vi "Write Resource Name.vi"(8 "error in (no error)":errorcluster, 10 "Resource Name":refnum<k15>, 11 "Power Meter in":refnum<class "Power Meter.lvclass">) -> (0 "error out":errorcluster, 3 "Power Meter out":refnum<class "Power Meter.lvclass">)   [LabVIEW 2023, in "NI-568x RF Power Meter.lvlib" / "Power Meter.lvclass"]
uses:
  Power Meter.lvclass
  Power Meter.lvclass/Power Meter.ctl
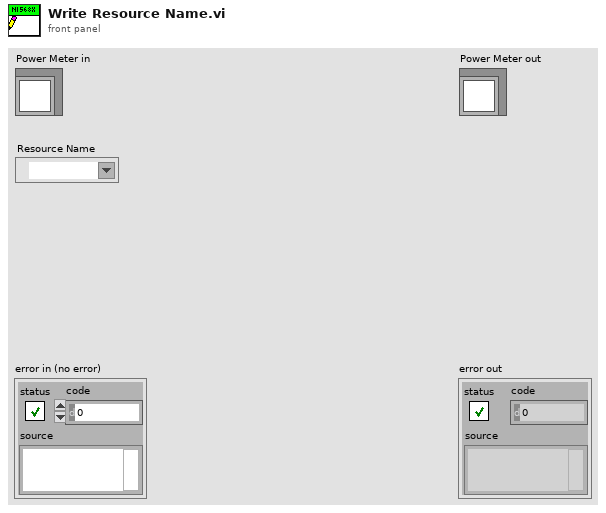
[diagram p1: front panel]
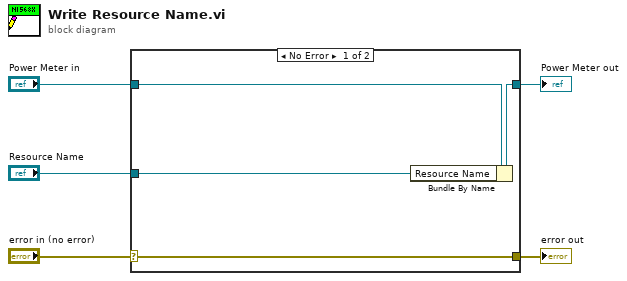
[diagram p0: block diagram]
diagram:
  n1 = case shown="No Error" "error in (no error)" {
    selector: "error in (no error)" -> [w9 w10]
    tunnel: [w9 w10] -> w4
    tunnel: [w7 w11] -> w2
    tunnel: "Power Meter in" -> [w8 w11]
    tunnel: "Resource Name" -> [w6 _]
    frame No Error {
      n2 = Bundle By Name(cluster=w8, "Resource Name"=w6) -> (w7:refnum<class "Power Meter.lvclass">)
    }
    frame Error {
    }
  }
  "error out" <- w4
  "Power Meter out" <- w2
